vi "Set Expires.vi"(8 "error in (no error)":errorcluster, 10 "Expires":timestamp, 11 "Cookie in":refnum<class "Cookie.lvclass">) -> (0 "error out":errorcluster, 3 "Cookie out":refnum<class "Cookie.lvclass">)   [LabVIEW 2020, in "HTTP Utils.lvlib" / "Cookie.lvclass"]
uses:
  Cookie.lvclass
  Cookie.lvclass/Cookie.ctl
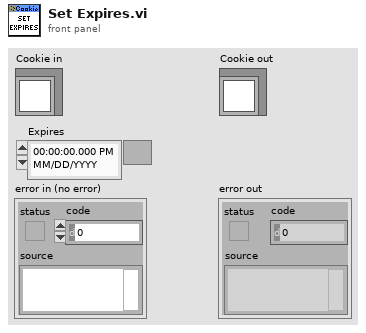
[diagram p1: front panel]
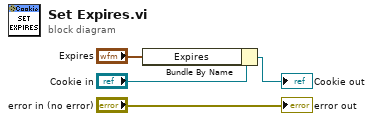
[diagram p0: block diagram]
diagram:
  n1 = Bundle By Name(cluster="Cookie in", "Expires"="Expires") -> (→"Cookie out":refnum<class "Cookie.lvclass">)
  "error out" <- "error in (no error)"
